vi "APC_9049_PressureAnalytics.vi"(4 "FilterCoefs":T1={"IIR LowPass"={"filter structure"=enum."IIR 2nd Order", "Reverse Coefficients"=[-1.7786317778245848, 0.8008026466657077], "Forward Coefficients"=[0.005542717210280682, 0.011085434420561363, 0.005542717210280682]}, "IIR HighPass"={"filter structure"=enum."IIR 2nd Order", "Reverse Coefficients"=[], "Forward Coefficients"=[]}} {"IIR LowPass"."Forward Coefficients" format="%.4f"; "IIR LowPass"."Reverse Coefficients" format="%.4f"}, 5 "AIdata [bar]":dbl[][](array[numeric])=array8x7200[57600 elements]) -> (1 "SyncCylPres [bar]":dbl[][](array[numeric]), 3 "9049_CalculatedVariablesRaster":dbl[](array[numeric]))   [LabVIEW 2020]
doc: "This example demonstrates the procedure required to apply different NI-DAQmx Custom Scales to each virtual channel in a task. A DAQmx Task Property Node (Functions >> NI Measurements >> DAQmx - Data Acquisition >> DAQmx Advanced Task Options) is used to obtain the task's virtual channels. A DAQmx Channel Property Node (Functions >> NI Measurements >> DAQmx - Data Acquisition) is then used to set the custom scale for each virtual channel in the task.\n\nThe \"DAQmx Create Scale\" VI creates a custom scale for each channel in the channel list. *Note, make sure your Minimum and Maximum channel parameters are consistent with the range the scale will create."
uses:
  controls/APC_CombustionMetrics.ctl
  controls/APC_PcylDiag.ctl
panel:
  in  "UsePcylDatabase":bool
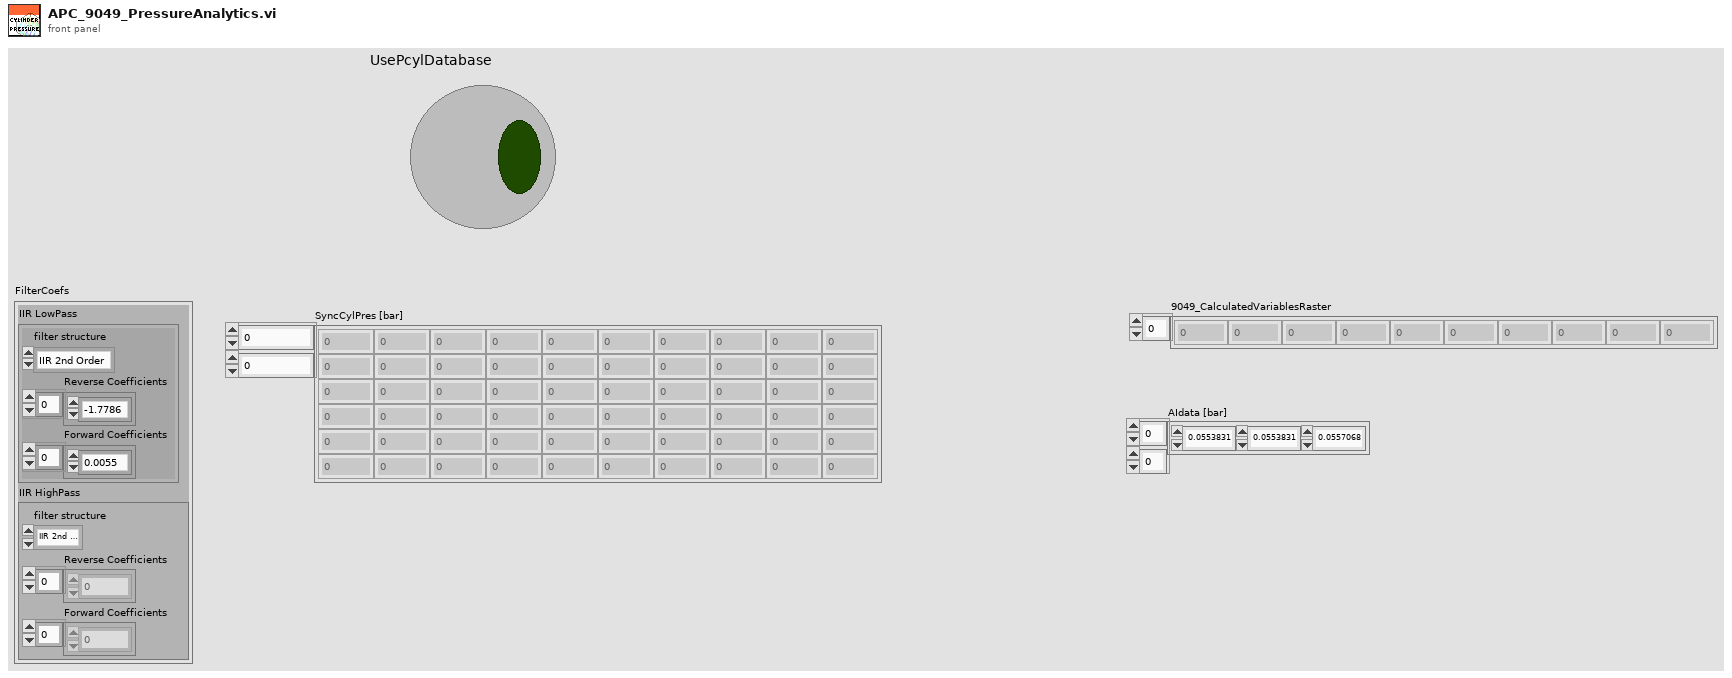
[diagram p1: front panel]
types:
  T1 = cluster{"IIR LowPass":cluster{"filter structure":enum32{"IIR 2nd Order", "IIR 4th Order"}, "Reverse Coefficients":dbl[], "Forward Coefficients":dbl[]}, "IIR HighPass":cluster{"filter structure":enum32{"IIR 2nd Order", "IIR 4th Order"}, "Reverse Coefficients":dbl[], "Forward Coefficients":dbl[]}}
  T2 = typedef "APC_CombustionMetrics.ctl" = cluster{"IMEPn [bar]":dbl[], "IMEPg [bar]":dbl[], "MAPO [bar/CAD]":dbl[], "maxQ [J]":dbl[], "CA10  [CADATDC]":dbl[], "CA50 [CADATDC]":dbl[], "CA90 [CADATDC]":dbl[], "Pmax [bar]":dbl[], "IMEPstd [bar]":dbl[], "CA03  [CADATDC]":dbl[], "CA97  [CADATDC]":dbl[], "CA10CA90 [CADATDC]":dbl[], "maxdpdCAD [bar/CAD]":dbl[], "kappa_comp [-]":dbl[], "kappa_exp [-]":dbl[], "PMEP [bar]":dbl[], "RI [-]":dbl[]}
  T3 = typedef "APC_PcylDiag.ctl" = cluster{"misfire from IMEP":bool[], "misfire self reg":bool[], "misfire cyl-to-cyl":bool[], "cyclic variability":bool[], "knock":bool[], "maximum pressure":bool[], "late combustion":bool[]}
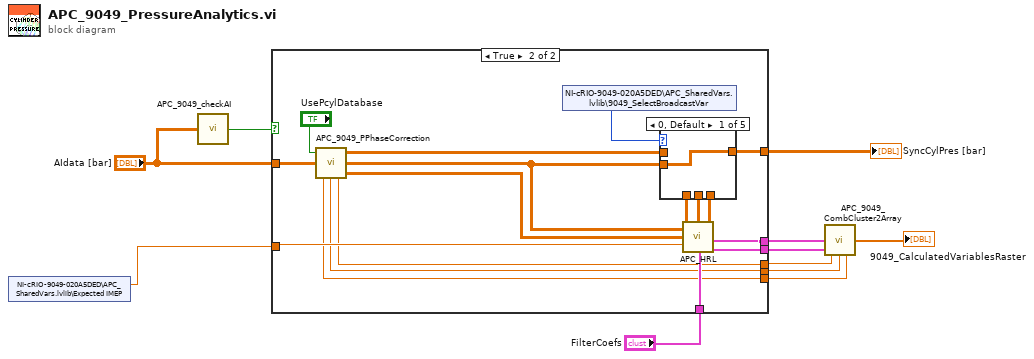
[diagram p0: block diagram]
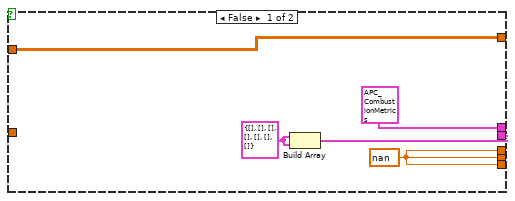
[diagram p2: hidden frame]
diagram:
  n1 = shared-variable "NI-cRIO-9049-020A5DED\\APC_SharedVars.lvlib\\Expected IMEP"() -> (w1:dbl)  [unwired: 1 in, 1 out]
  n2 = call "APC_9049_checkAI.vi"("AIdata [bar]"="AIdata [bar]") -> ("x = y?"=w4:bool)
  n3 = case shown="True" w4 {
    tunnel: [w12 w21] -> w10
    tunnel: "AIdata [bar]" -> [w15 w19]
    tunnel: "FilterCoefs" -> [_ w33]
    tunnel: [w12 w20] -> w9
    tunnel: w1 -> [_ w32]
    tunnel: [T2 {"IMEPn [bar]"=[nan, nan, nan, nan, nan, nan], "IMEPg [bar]"=[nan, nan, nan, nan, nan, nan], "MAPO [bar/CAD]"=[nan, nan, nan, nan, nan, nan], "maxQ [J]"=[nan, nan, nan, nan, nan, nan], "CA10  [CADATDC]"=[nan, nan, nan, nan, nan, nan], "CA50 [CADATDC]"=[nan, nan, nan, nan, nan, nan], "CA90 [CADATDC]"=[nan, nan, nan, nan, nan, nan], "Pmax [bar]"=[nan, nan, nan, nan, nan, nan], "IMEPstd [bar]"=[nan, nan, nan, nan, nan, nan], "CA03  [CADATDC]"=[nan, nan, nan, nan, nan, nan], "CA97  [CADATDC]"=[nan, nan, nan, nan, nan, nan], "CA10CA90 [CADATDC]"=[nan, nan, nan, nan, nan, nan], "maxdpdCAD [bar/CAD]"=[nan, nan, nan, nan, nan, nan], "kappa_comp [-]"=[nan, nan, nan, nan, nan, nan], "kappa_exp [-]"=[nan, nan, nan, nan, nan, nan], "PMEP [bar]"=[nan, nan, nan, nan, nan, nan], "RI [-]"=[nan, nan, nan, nan, nan, nan]} ("CombustionAnalysisClusterOut") w31] -> w6
    tunnel: [w15 w27] -> w7
    tunnel: [w13 w26] -> w5
    tunnel: [w12 w17] -> w2
    frame False {
      w14 = T3 {"misfire from IMEP"=[], "misfire self reg"=[], "misfire cyl-to-cyl"=[], "cyclic variability"=[], "knock"=[], "maximum pressure"=[], "late combustion"=[]} ("PcylDiag")
      w12 = nan ("mean")
      n4 = Build Array(w14, w14) -> (w13:T3[])
    }
    frame True {
      n5 = call "APC_9049_PPhaseCorrection.vi"("UsePcylDatabase"="UsePcylDatabase", "AIdata [bar]"=w19) -> ("SystemP [bar]"=w21:dbl, "PrechamberPeakDiff [bar]"=w17:dbl, "ExhaustP [bar]"=w20:dbl, "RawPcyl [bar]"=w24:dbl[][], "PhaseCompPcyl [bar]"=w23:dbl[][], "PhaseCompPexh [bar]"=w22:dbl[][])
      n6 = shared-variable "NI-cRIO-9049-020A5DED\\APC_SharedVars.lvlib\\9049_SelectBroadcastVar"() -> (w25:u8)  [unwired: 1 in, 1 out]
      n7 = call "APC_HRL.vi"("Pcyl"=w23, "exhaust pressure"=w22, "FilterCoefs"=w33, "Expected IMEP"=w32) -> ("LPfilt Pcyl"=w29:dbl[][], "HRL [J]"=w28:dbl[][], "CombustionAnalysisCluster"=w31:T2, "HPfilt Pcyl"=w30:dbl[][], "PcylDiagWarningsAndErrors"=w26:T3[])
      n8 = case shown="0, Default" w25 {
        tunnel: w23 -> [w34 _ _ _ _]
        tunnel: [w34 w35 w36 w37 w38] -> w27
        tunnel: w24 -> [_ w35 _ _ _]
        tunnel: w30 -> [_ _ _ w37 _]
        tunnel: w29 -> [_ _ w36 _ _]
        tunnel: w28 -> [_ _ _ _ w38]
        frame 0, Default {
        }
        frame 4 {
        }
        frame 1 {
        }
        frame 2 {
        }
        frame 3 {
        }
      }
    }
  }
  "SyncCylPres [bar]" <- w7
  n9 = call "APC_9049_CombCluster2Array.vi"("SystemPressure"=w10, "CombustionAnalysisCluster"=w6, "ExhPressure"=w9, "PcylDiag"=w5, "PrechamberPeakPdiff"=w2) -> ("9049_CalculatedVariablesRaster"=→"9049_CalculatedVariablesRaster":dbl[])
